vi "Tic-Tac-Toe.vi"() -> ()   [LabVIEW 2014]
uses:
  Downloads/TTT2011/Symbol.ctl
panel:
  in  "stop":bool
  out "Turn":string
  in  "Ring 9":u16(ring)
  in  "Ring 8":u16(ring)
  in  "Ring 7":u16(ring)
  in  "Ring 6":u16(ring)
  in  "Ring 5":u16(ring)
  in  "Ring 4":u16(ring)
  in  "Ring 3":u16(ring)
  in  "Ring 2":u16(ring)
  in  "Ring 1":u16(ring)
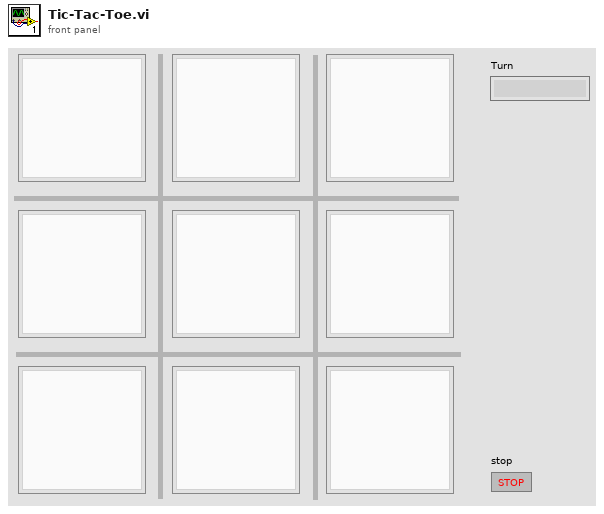
[diagram p1: front panel]
types:
  T1 = typedef "Symbol.ctl" = u16
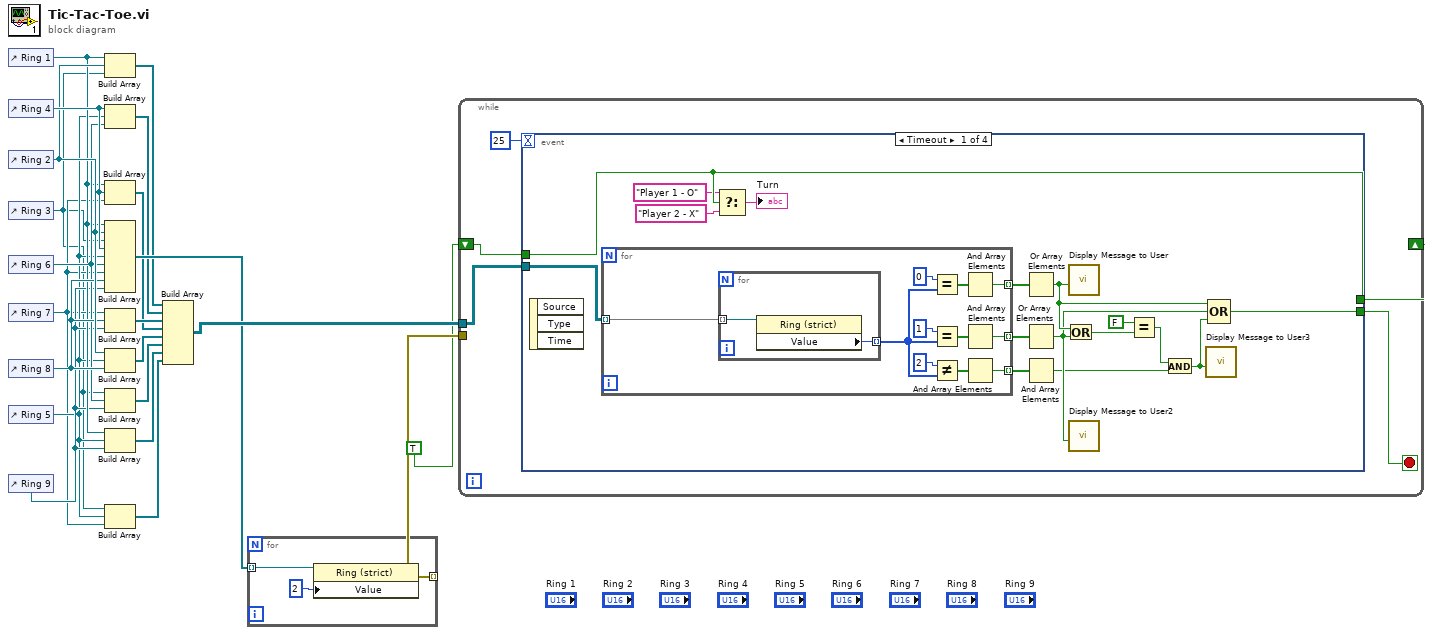
[diagram p0: block diagram]
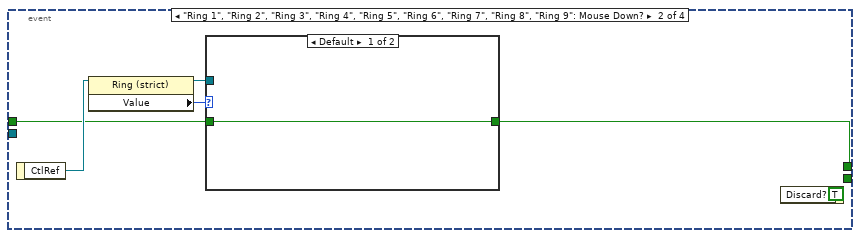
[diagram p2: hidden frame]
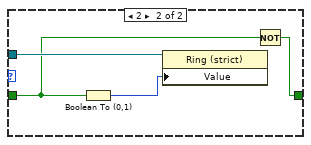
[diagram p3: hidden frame]
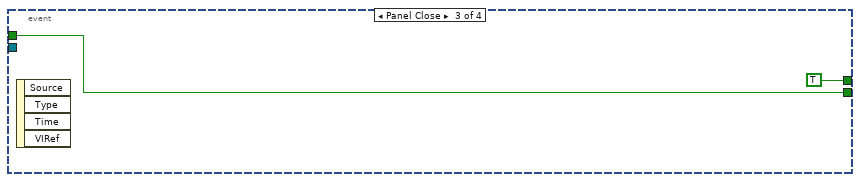
[diagram p4: hidden frame]
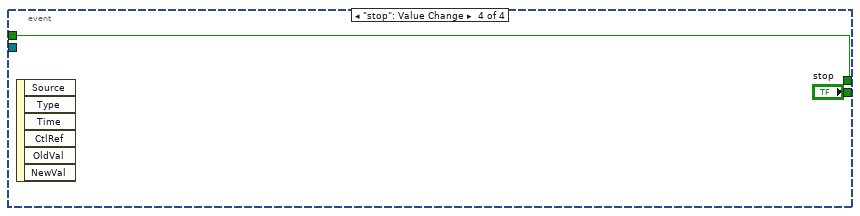
[diagram p5: hidden frame]
diagram:
  n1 = control-ref of="Ring 1"() -> (w6:refnum<vi>)
  n2 = control-ref of="Ring 4"() -> (w13:refnum<vi>)
  n3 = control-ref of="Ring 2"() -> (w11:refnum<vi>)
  n4 = control-ref of="Ring 3"() -> (w1:refnum<vi>)
  n5 = control-ref of="Ring 6"() -> (w8:refnum<vi>)
  n6 = control-ref of="Ring 7"() -> (w2:refnum<vi>)
  n7 = control-ref of="Ring 8"() -> (w10:refnum<vi>)
  n8 = control-ref of="Ring 5"() -> (w3:refnum<vi>)
  n9 = control-ref of="Ring 9"() -> (w4:refnum<vi>)
  n10 = Build Array(w6, w11, w1) -> (w17:refnum<vi>[])
  n11 = Build Array(w13, w3, w8) -> (w16:refnum<vi>[])
  n12 = Build Array(w6, w13, w2) -> (w14:refnum<vi>[])
  n13 = Build Array(w6, w11, w1, w13, w3, w8, w2, w10, w4) -> (w18:refnum<vi>[])
  n14 = Build Array(w2, w10, w4) -> (w15:refnum<vi>[])
  n15 = Build Array(w11, w3, w10) -> (w12:refnum<vi>[])
  n16 = Build Array(w1, w8, w4) -> (w9:refnum<vi>[])
  n17 = Build Array(w6, w3, w4) -> (w7:refnum<vi>[])
  n18 = Build Array(w1, w3, w2) -> (w5:refnum<vi>[])
  n19 = Build Array(w17, w16, w15, w14, w12, w9, w7, w5) -> (w21:refnum<vi>[][])
  n20 = for {
    tunnel: [w23] -> w20 mode=indexing
    tunnel: w18 -> [w22] mode=indexing
    n21 = property class="Ring (strict)"(reference=w22, "Value"=T1 2) -> (error out=w23:errorcluster)  [unwired: 1 in, 1 out]
  }
  n22 = while {
    tunnel: w21 -> [w28]
    tunnel: w20 -> [_]
    shift-right: [w25] -> _
    shift-left: TRUE -> [w26]
    stop <- w27 stop-if-true
    n23 = event shown="[0] Timeout" {
      selector: _ -> [_ _ _ _]
      dyn-events: _ -> [_ _ _ _]
      timeout: 25 -> [_ _ _ _]
      tunnel: w28 -> [w45 _ _ _]
      tunnel: [w42 _ w71 "stop"] -> w27
      tunnel: [w40 w61 TRUE w72] -> w25
      tunnel: w26 -> [w40 w62 w71 w72]
      event Timeout {
        n24 = event-data() -> ()  [unwired: 1 in, 3 out]
        n25 = for {
          tunnel: w45 -> [w56] mode=indexing
          tunnel: [w53] -> w44 mode=indexing
          tunnel: [w52] -> w43 mode=indexing
          tunnel: [w46] -> w37 mode=indexing
          n26 = for {
            tunnel: w56 -> [w57] mode=indexing
            tunnel: [w58] -> w49 mode=indexing
            n27 = property class="Ring (strict)"(reference=w57) -> ("Value"=w58:u16)  [unwired: 1 in, 2 out]
          }
          n28 = Equal?(x=0 ("Value"), y=w49) -> (x = y?=w55:bool[])
          n29 = Equal?(x=1 ("Value"), y=w49) -> (x = y?=w54:bool[])
          n30 = Not Equal?(x=2, y=w49) -> (x != y?=w47:bool[])
          n31 = And Array Elements(Boolean array=w55) -> (logical AND=w53:bool)
          n32 = And Array Elements(Boolean array=w54) -> (logical AND=w52:bool)
          n33 = And Array Elements(Boolean array=w47) -> (logical AND=w46:bool)
        }
        n34 = Select(t="Player 1 - O", s=w40, f="Player 2 - X") -> (s? t:f=→"Turn":string)
        n35 = Or Array Elements(Boolean array=w44) -> (logical OR=w36:bool)
        n36 = Or Array Elements(Boolean array=w43) -> (logical OR=w35:bool)
        n37 = And Array Elements(Boolean array=w37) -> (logical AND=w31:bool)
        n38 = Or(x=w36, y=w35) -> (x .or. y?=w34:bool)
        n39 = call "Display Message to User"("Enable"=w36) -> ()  [unwired: 9 in, 2 out]
        n40 = call "Display Message to User2"("Enable"=w35) -> ()  [unwired: 9 in, 2 out]
        n41 = Equal?(x=FALSE, y=w34) -> (x = y?=w32:bool)
        n42 = And(x=w32, y=w31) -> (x .and. y?=w30:bool)
        n43 = call "Display Message to User3"("Enable"=w30) -> ()  [unwired: 9 in, 2 out]
        n44 = Compound Arithmetic op=OR(w36, w35, w30) -> (w42:bool)
      }
      event "Ring 1", "Ring 2", "Ring 3", "Ring 4", "Ring 5", "Ring 6", "Ring 7", "Ring 8", "Ring 9": Mouse Down? {
        n45 = event-data() -> ("CtlRef"=w64:refnum<vi>)  [unwired: 1 in]
        n46 = property class="Ring (strict)"(reference=w64) -> (reference out=w60:refnum<vi>, "Value"=w63:u16)  [unwired: 1 in, 1 out]
        n47 = case shown="Default" w63 {
          tunnel: w62 -> [w65 w67]
          tunnel: [w65 w66] -> w61
          tunnel: w60 -> [_ w69]
          frame Default {
          }
          frame 2 {
            n48 = Boolean To (0,1)(Boolean=w67) -> (0, 1=w68:i16)
            n49 = property class="Ring (strict)"(reference=w69, "Value"=w68) -> ()  [unwired: 1 in, 2 out]
            n50 = Not(x=w67) -> (.not. x?=w66:bool)
          }
        }
        n51 = event-data("Discard?"=TRUE) -> ()  [unwired: 1 in, 1 out]
      }
      event Panel Close {
        n52 = event-data() -> ()  [unwired: 1 in, 4 out]
      }
      event "stop": Value Change {
        n53 = event-data() -> ()  [unwired: 1 in, 6 out]
      }
    }
  }
